vi "加标回收调试界面.vi"() -> ()   [LabVIEW 2016, in "质控单元V4.lvlib"]
uses:
  <vilib>/Utility/miscctls.llb/LVPointTypeDef.ctl
  <vilib>/Utility/miscctls.llb/LVPositionTypeDef.ctl
panel:
  in  "关闭":bool
  out "流程 2":T1 {"进样流程"."进样流程-进样"."步骤二："."功能" items=["加标", "进样", "排液", "搅拌", "定量", "延时"]; "进样流程"."进样流程-进样"."步骤一："."功能" items=["加标", "进样", "排液", "搅拌", "定量", "延时"]; "进样流程"."进样流程-进样"."步骤四："."功能" items=["加标", "进样", "排液", "搅拌", "定量", "延时"]; "进样流程"."进样流程-进样"."步骤三："."功能" items=["加标", "进样", "排液", "搅拌", "定量", "延时"]; "进样流程"."进样流程-进样"."步骤六："."功能" items=["加标", "进样", "排液", "搅拌", "定量", "延时"]; "进样流程"."进样流程-进样"."步骤五："."功能" items=["加标", "进样", "排液", "搅拌", "定量", "延时"]; "进样流程"."进样流程-进样"."步骤八："."功能" items=["加标", "进样", "排液", "搅拌", "定量", "延时"]; "进样流程"."进样流程-进样"."步骤七："."功能" items=["加标", "进样", "排液", "搅拌", "定量", "延时"]; "进样流程"."进样流程-进样"."步骤十："."功能" items=["加标", "进样", "排液", "搅拌", "定量", "延时"]; "进样流程"."进样流程-进样"."步骤九："."功能" items=["加标", "进样", "排液", "搅拌", "定量", "延时"]; "进样流程"."进样流程-润洗"."步骤二："."功能" items=["加标", "进样", "排液", "搅拌", "定量", "延时"]; "进样流程"."进样流程-润洗"."步骤一："."功能" items=["加标", "进样", "排液", "搅拌", "定量", "延时"]; "进样流程"."进样流程-润洗"."步骤四："."功能" items=["加标", "进样", "排液", "搅拌", "定量", "延时"]; "进样流程"."进样流程-润洗"."步骤三："."功能" items=["加标", "进样", "排液", "搅拌", "定量", "延时"]; "进样流程"."进样流程-润洗"."步骤六："."功能" items=["加标", "进样", "排液", "搅拌", "定量", "延时"]; "进样流程"."进样流程-润洗"."步骤五："."功能" items=["加标", "进样", "排液", "搅拌", "定量", "延时"]; "进样流程"."进样流程-润洗"."步骤八："."功能" items=["加标", "进样", "排液", "搅拌", "定量", "延时"]; "进样流程"."进样流程-润洗"."步骤七："."功能" items=["加标", "进样", "排液", "搅拌", "定量", "延时"]; "进样流程"."进样流程-润洗"."步骤十："."功能" items=["加标", "进样", "排液", "搅拌", "定量", "延时"]; "进样流程"."进样流程-润洗"."步骤九："."功能" items=["加标", "进样", "排液", "搅拌", "定量", "延时"]; "排液流程"."步骤二："."功能" items=["加标", "进样", "排液", "搅拌", "定量", "延时"]; "排液流程"."步骤一："."功能" items=["加标", "进样", "排液", "搅拌", "定量", "延时"]; "排液流程"."步骤四："."功能" items=["加标", "进样", "排液", "搅拌", "定量", "延时"]; "排液流程"."步骤三："."功能" items=["加标", "进样", "排液", "搅拌", "定量", "延时"]; "排液流程"."步骤六："."功能" items=["加标", "进样", "排液", "搅拌", "定量", "延时"]; "排液流程"."步骤五："."功能" items=["加标", "进样", "排液", "搅拌", "定量", "延时"]; "排液流程"."步骤八："."功能" items=["加标", "进样", "排液", "搅拌", "定量", "延时"]; "排液流程"."步骤七："."功能" items=["加标", "进样", "排液", "搅拌", "定量", "延时"]; "排液流程"."步骤十："."功能" items=["加标", "进样", "排液", "搅拌", "定量", "延时"]; "排液流程"."步骤九："."功能" items=["加标", "进样", "排液", "搅拌", "定量", "延时"]; "加标流程"."加标流程-加标"."步骤二："."功能" items=["加标", "进样", "排液", "搅拌", "定量", "延时"]; "加标流程"."加标流程-加标"."步骤一："."功能" items=["加标", "进样", "排液", "搅拌", "定量", "延时"]; "加标流程"."加标流程-加标"."步骤四："."功能" items=["加标", "进样", "排液", "搅拌", "定量", "延时"]; "加标流程"."加标流程-加标"."步骤三："."功能" items=["加标", "进样", "排液", "搅拌", "定量", "延时"]; "加标流程"."加标流程-加标"."步骤六："."功能" items=["加标", "进样", "排液", "搅拌", "定量", "延时"]; "加标流程"."加标流程-加标"."步骤五："."功能" items=["加标", "进样", "排液", "搅拌", "定量", "延时"]; "加标流程"."加标流程-加标"."步骤八："."功能" items=["加标", "进样", "排液", "搅拌", "定量", "延时"]; "加标流程"."加标流程-加标"."步骤七："."功能" items=["加标", "进样", "排液", "搅拌", "定量", "延时"]; "加标流程"."加标流程-加标"."步骤十："."功能" items=["加标", "进样", "排液", "搅拌", "定量", "延时"]; "加标流程"."加标流程-加标"."步骤九："."功能" items=["加标", "进样", "排液", "搅拌", "定量", "延时"]; "加标流程"."加标流程-定量"."步骤二："."功能" items=["加标", "进样", "排液", "搅拌", "定量", "延时"]; "加标流程"."加标流程-定量"."步骤一："."功能" items=["加标", "进样", "排液", "搅拌", "定量", "延时"]; "加标流程"."加标流程-定量"."步骤四："."功能" items=["加标", "进样", "排液", "搅拌", "定量", "延时"]; "加标流程"."加标流程-定量"."步骤三："."功能" items=["加标", "进样", "排液", "搅拌", "定量", "延时"]; "加标流程"."加标流程-定量"."步骤六："."功能" items=["加标", "进样", "排液", "搅拌", "定量", "延时"]; "加标流程"."加标流程-定量"."步骤五："."功能" items=["加标", "进样", "排液", "搅拌", "定量", "延时"]; "加标流程"."加标流程-定量"."步骤八："."功能" items=["加标", "进样", "排液", "搅拌", "定量", "延时"]; "加标流程"."加标流程-定量"."步骤七："."功能" items=["加标", "进样", "排液", "搅拌", "定量", "延时"]; "加标流程"."加标流程-定量"."步骤十："."功能" items=["加标", "进样", "排液", "搅拌", "定量", "延时"]; "加标流程"."加标流程-定量"."步骤九："."功能" items=["加标", "进样", "排液", "搅拌", "定量", "延时"]; "加标流程"."加标流程-进样"."步骤二："."功能" items=["加标", "进样", "排液", "搅拌", "定量", "延时"]; "加标流程"."加标流程-进样"."步骤一："."功能" items=["加标", "进样", "排液", "搅拌", "定量", "延时"]; "加标流程"."加标流程-进样"."步骤四："."功能" items=["加标", "进样", "排液", "搅拌", "定量", "延时"]; "加标流程"."加标流程-进样"."步骤三："."功能" items=["加标", "进样", "排液", "搅拌", "定量", "延时"]; "加标流程"."加标流程-进样"."步骤六："."功能" items=["加标", "进样", "排液", "搅拌", "定量", "延时"]; "加标流程"."加标流程-进样"."步骤五："."功能" items=["加标", "进样", "排液", "搅拌", "定量", "延时"]; "加标流程"."加标流程-进样"."步骤八："."功能" items=["加标", "进样", "排液", "搅拌", "定量", "延时"]; "加标流程"."加标流程-进样"."步骤七："."功能" items=["加标", "进样", "排液", "搅拌", "定量", "延时"]; "加标流程"."加标流程-进样"."步骤十："."功能" items=["加标", "进样", "排液", "搅拌", "定量", "延时"]; "加标流程"."加标流程-进样"."步骤九："."功能" items=["加标", "进样", "排液", "搅拌", "定量", "延时"]; "加标流程"."加标流程-润洗"."步骤二："."功能" items=["加标", "进样", "排液", "搅拌", "定量", "延时"]; "加标流程"."加标流程-润洗"."步骤一："."功能" items=["加标", "进样", "排液", "搅拌", "定量", "延时"]; "加标流程"."加标流程-润洗"."步骤四："."功能" items=["加标", "进样", "排液", "搅拌", "定量", "延时"]; "加标流程"."加标流程-润洗"."步骤三："."功能" items=["加标", "进样", "排液", "搅拌", "定量", "延时"]; "加标流程"."加标流程-润洗"."步骤六："."功能" items=["加标", "进样", "排液", "搅拌", "定量", "延时"]; "加标流程"."加标流程-润洗"."步骤五："."功能" items=["加标", "进样", "排液", "搅拌", "定量", "延时"]; "加标流程"."加标流程-润洗"."步骤八："."功能" items=["加标", "进样", "排液", "搅拌", "定量", "延时"]; "加标流程"."加标流程-润洗"."步骤七："."功能" items=["加标", "进样", "排液", "搅拌", "定量", "延时"]; "加标流程"."加标流程-润洗"."步骤十："."功能" items=["加标", "进样", "排液", "搅拌", "定量", "延时"]; "加标流程"."加标流程-润洗"."步骤九："."功能" items=["加标", "进样", "排液", "搅拌", "定量", "延时"]; "加标润洗流程"."步骤二："."功能" items=["加标", "进样", "排液", "搅拌", "定量", "延时"]; "加标润洗流程"."步骤一："."功能" items=["加标", "进样", "排液", "搅拌", "定量", "延时"]; "加标润洗流程"."步骤四："."功能" items=["加标", "进样", "排液", "搅拌", "定量", "延时"]; "加标润洗流程"."步骤三："."功能" items=["加标", "进样", "排液", "搅拌", "定量", "延时"]; "加标润洗流程"."步骤六："."功能" items=["加标", "进样", "排液", "搅拌", "定量", "延时"]; "加标润洗流程"."步骤五："."功能" items=["加标", "进样", "排液", "搅拌", "定量", "延时"]; "加标润洗流程"."步骤八："."功能" items=["加标", "进样", "排液", "搅拌", "定量", "延时"]; "加标润洗流程"."步骤七："."功能" items=["加标", "进样", "排液", "搅拌", "定量", "延时"]; "加标润洗流程"."步骤十："."功能" items=["加标", "进样", "排液", "搅拌", "定量", "延时"]; "加标润洗流程"."步骤九："."功能" items=["加标", "进样", "排液", "搅拌", "定量", "延时"]; "水样润洗流程"."步骤二："."功能" items=["加标", "进样", "排液", "搅拌", "定量", "延时"]; "水样润洗流程"."步骤一："."功能" items=["加标", "进样", "排液", "搅拌", "定量", "延时"]; "水样润洗流程"."步骤四："."功能" items=["加标", "进样", "排液", "搅拌", "定量", "延时"]; "水样润洗流程"."步骤三："."功能" items=["加标", "进样", "排液", "搅拌", "定量", "延时"]; "水样润洗流程"."步骤六："."功能" items=["加标", "进样", "排液", "搅拌", "定量", "延时"]; "水样润洗流程"."步骤五："."功能" items=["加标", "进样", "排液", "搅拌", "定量", "延时"]; "水样润洗流程"."步骤八："."功能" items=["加标", "进样", "排液", "搅拌", "定量", "延时"]; "水样润洗流程"."步骤七："."功能" items=["加标", "进样", "排液", "搅拌", "定量", "延时"]; "水样润洗流程"."步骤十："."功能" items=["加标", "进样", "排液", "搅拌", "定量", "延时"]; "水样润洗流程"."步骤九："."功能" items=["加标", "进样", "排液", "搅拌", "定量", "延时"]}
  in  "请选择模块":T2(radio)=enum."氨氮"
  in  "关于":bool
  in  "Tab Control 4":enum32{"参数"}(tab)
  out "剩余时间":string
  out "当前步骤":string
  out "当前流程":string
  out "告警状态":string
  out "液位状态":string
  out "运行状态":string
  out "通讯状态":bool caption="状态"
  in  "Tab Control 3":enum32{"参数设置", "单步调试", "流程写入"}(tab)
  in  "加标体积读取":bool
  in  "加标体积写入":bool
  in  "蠕动泵参数读取":bool
  in  "蠕动泵参数写入":bool
  in  "B":sgl
  in  "K":sgl
  in  "蠕动泵最小频率(Hz)":sgl
  in  "蠕动泵最大频率(Hz)":sgl
  in  "加标体积(mL)":sgl
  in  "注射泵系数读取":bool
  in  "注射泵系数写入":bool
  in  "质控类型":u16(ring) items=["固定站", "一体站"]
  in  "质控类型读取":bool
  in  "质控类型写入":bool
  in  "蠕动泵2停止":bool
  in  "蠕动泵2正转":bool
  in  "蠕动泵2反转":bool
  in  "蠕动泵1停止":bool
  in  "蠕动泵1正转":bool
  in  "蠕动泵1反转":bool
  in  "三通阀2打开":bool
  in  "三通阀2关闭":bool
  in  "三通阀1打开":bool
  in  "三通阀1关闭":bool
  in  "注射泵复位":bool
  in  "注射泵暂停":bool
  in  "注射泵注入量":sgl=1000.0 min=0 max=1000 format="%u μL"
  in  "注射泵注出量":sgl=1000.0 min=0 max=1000 format="%u μL"
  in  "注射泵注出":bool
  in  "注射泵注入":bool
  in  "三通阀打开":bool
  in  "三通阀关闭":bool
  in  "流程保存":bool
  in  "流程加载":bool
  in  "流程写入":bool
  in  "流程读取":bool
  in  "子流程":u16(ring) items=["润洗"]
  in  "主流程":T3(ring)
  in  "流程":T4 {"步骤二："."功能" items=["加标", "进样", "排液", "搅拌", "定量", "延时"]; "步骤四："."功能" items=["加标", "进样", "排液", "搅拌", "定量", "延时"]; "步骤六："."功能" items=["加标", "进样", "排液", "搅拌", "定量", "延时"]; "步骤八："."功能" items=["加标", "进样", "排液", "搅拌", "定量", "延时"]; "步骤十："."功能" items=["加标", "进样", "排液", "搅拌", "定量", "延时"]; "步骤一："."功能" items=["加标", "进样", "排液", "搅拌", "定量", "延时"]; "步骤三："."功能" items=["加标", "进样", "排液", "搅拌", "定量", "延时"]; "步骤五："."功能" items=["加标", "进样", "排液", "搅拌", "定量", "延时"]; "步骤七："."功能" items=["加标", "进样", "排液", "搅拌", "定量", "延时"]; "步骤九："."功能" items=["加标", "进样", "排液", "搅拌", "定量", "延时"]}
  in  "Tab Control 2":enum32{"参数"}(tab)
  in  "启动水样润洗流程":bool
  in  "启动进样流程":bool
  in  "启动加标流程":bool
  in  "启动排液流程":bool
  in  "停止所有流程":bool
  in  "启动加标润洗流程":bool
  in  "组合操作停止":bool
  in  "组合操作定量":bool
  in  "组合操作进空气":bool
  in  "组合操作排废液":bool
  in  "组合操作进水样":bool
  in  "清除告警":bool
  # "仪器状态"
  # "柱塞泵泵系数"
  # "柱塞泵"
  # "三通阀"
  # "泵阀"
  # "三通阀1"
  # "三通阀2"
  # "蠕动泵1"
  # "蠕动泵2"
  # "仪器端："
  # "PC端："
  # "组合步骤"
  # "测试流程"
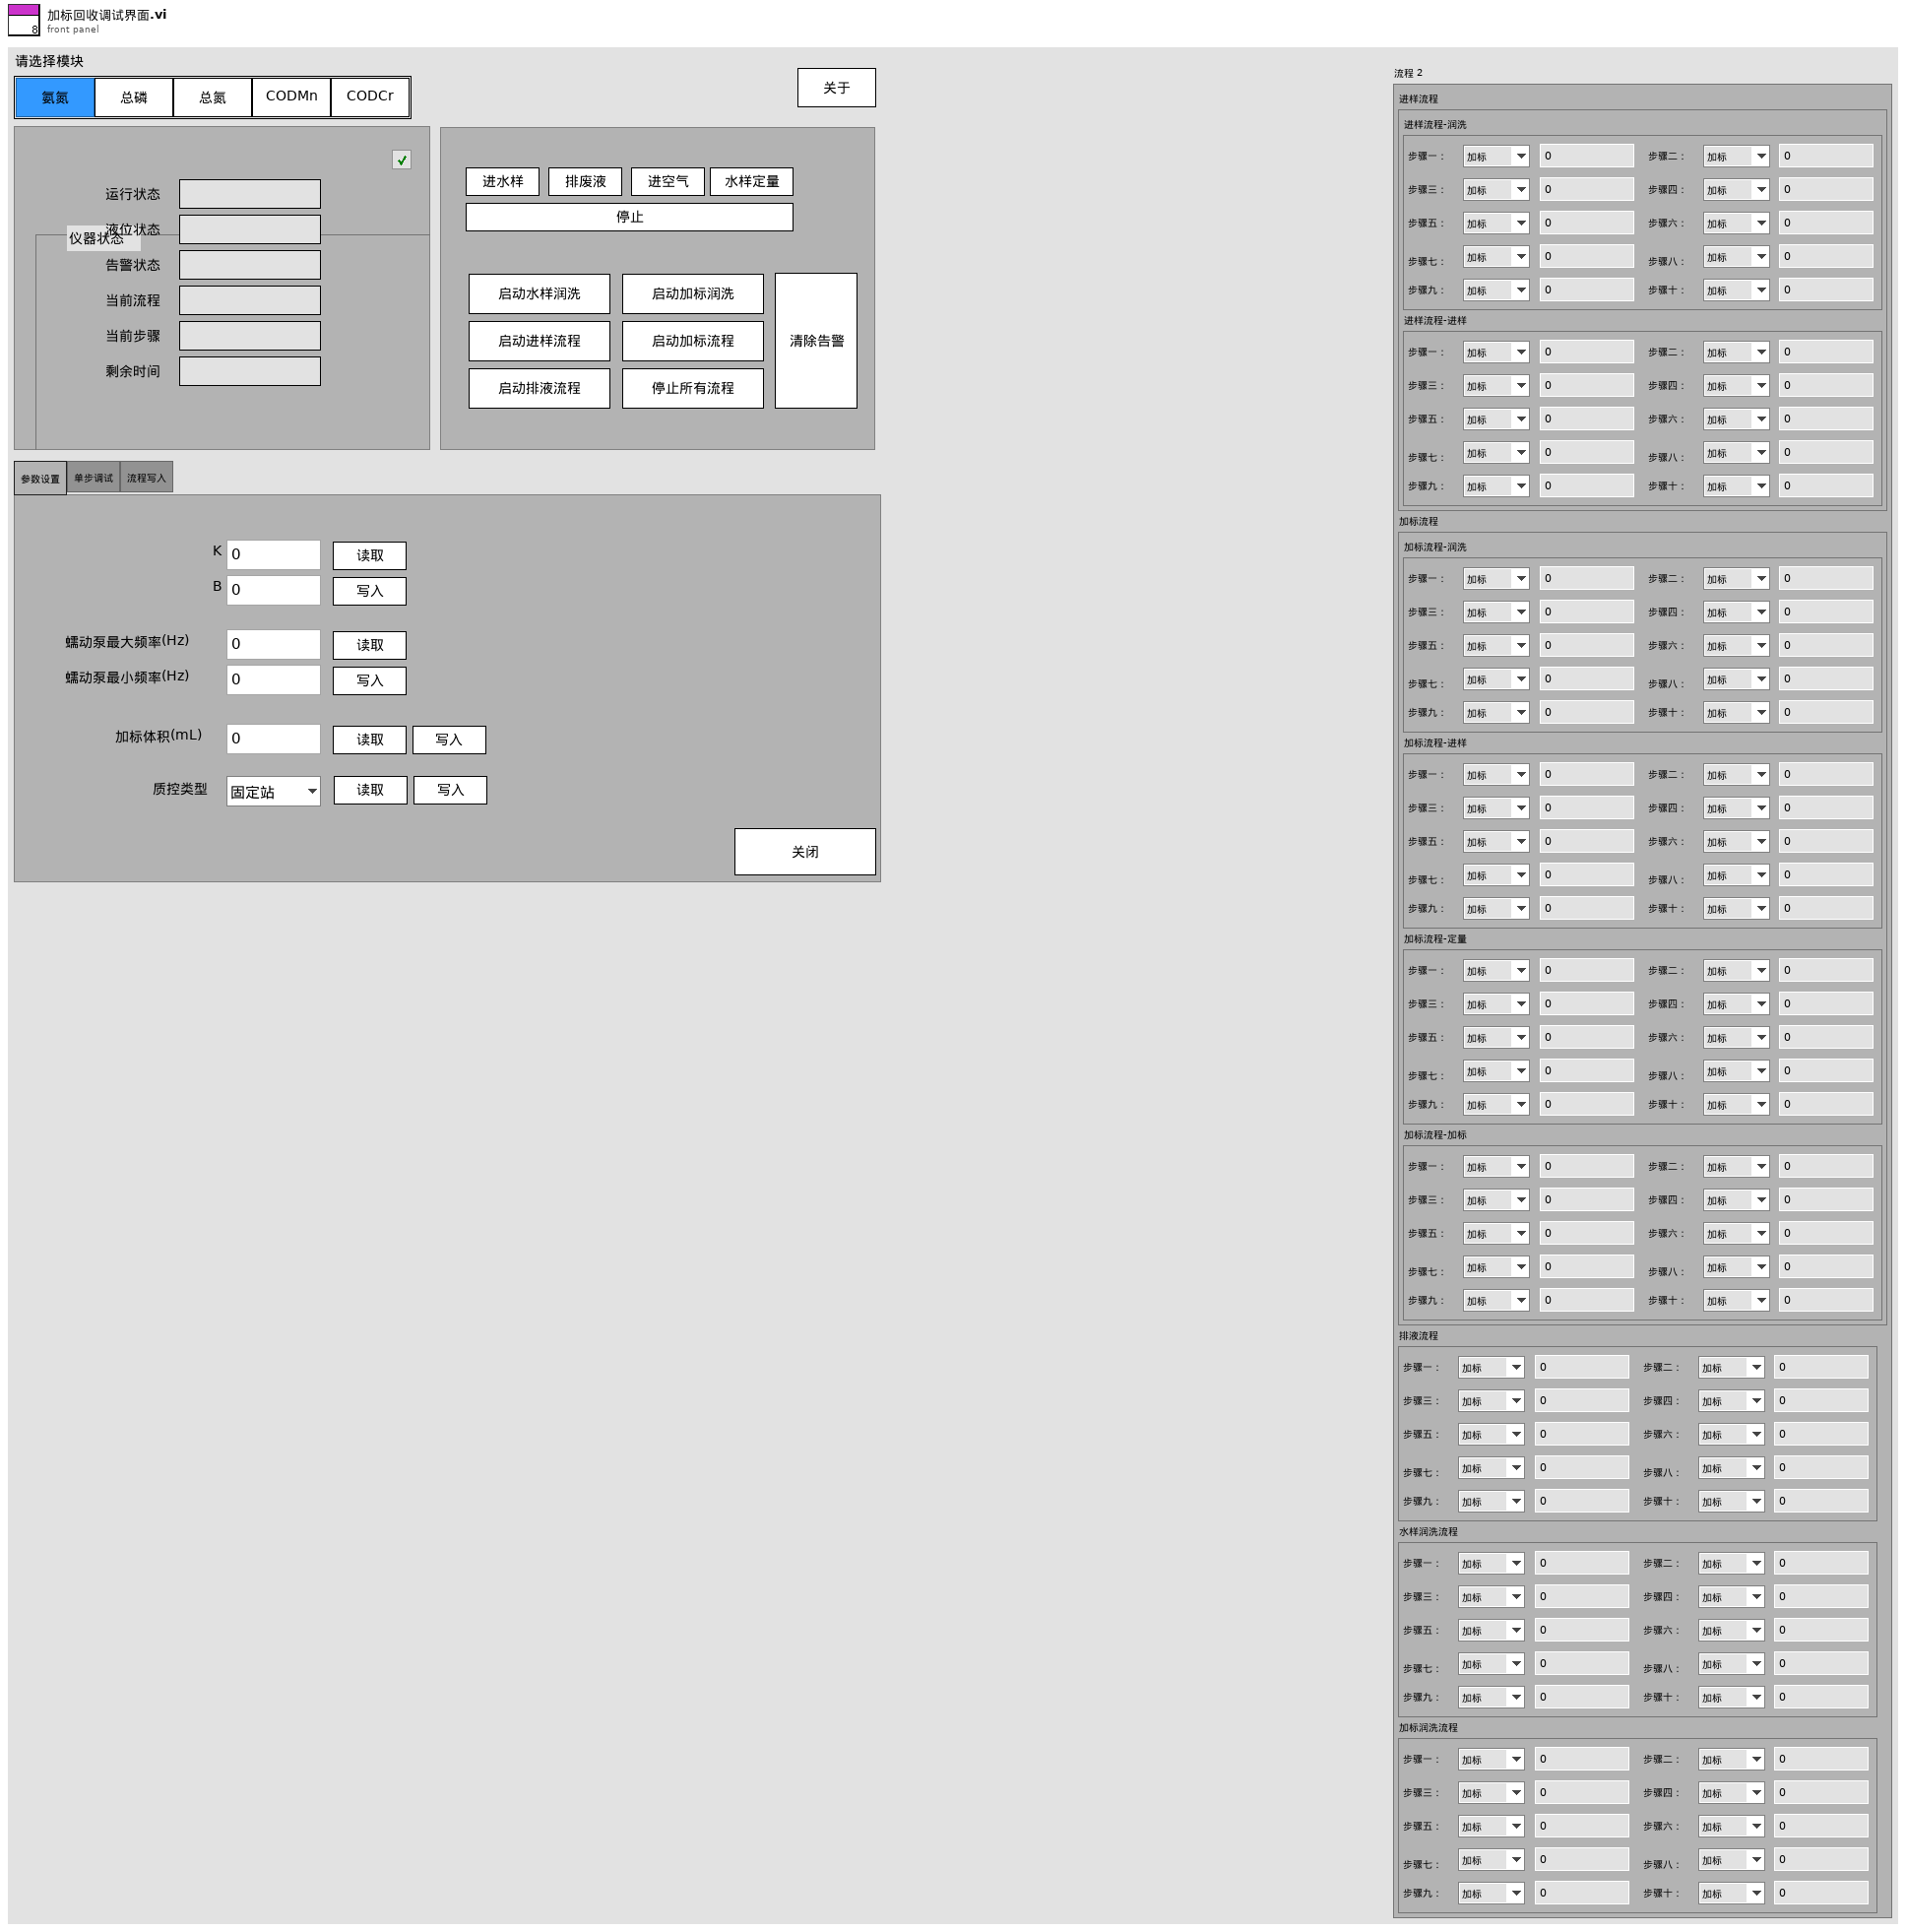
[diagram p1: front panel]
types:
  T1 = cluster{"进样流程":cluster{"进样流程-润洗":cluster{"步骤一：":cluster{"功能":u16, "值":sgl}, "步骤二：":cluster{"功能":u16, "值":sgl}, "步骤三：":cluster{"功能":u16, "值":sgl}, "步骤四：":cluster{"功能":u16, "值":sgl}, "步骤五：":cluster{"功能":u16, "值":sgl}, "步骤六：":cluster{"功能":u16, "值":sgl}, "步骤七：":cluster{"功能":u16, "值":sgl}, "步骤八：":cluster{"功能":u16, "值":sgl}, "步骤九：":cluster{"功能":u16, "值":sgl}, "步骤十：":cluster{"功能":u16, "值":sgl}}, "进样流程-进样":cluster{"步骤一：":cluster{"功能":u16, "值":sgl}, "步骤二：":cluster{"功能":u16, "值":sgl}, "步骤三：":cluster{"功能":u16, "值":sgl}, "步骤四：":cluster{"功能":u16, "值":sgl}, "步骤五：":cluster{"功能":u16, "值":sgl}, "步骤六：":cluster{"功能":u16, "值":sgl}, "步骤七：":cluster{"功能":u16, "值":sgl}, "步骤八：":cluster{"功能":u16, "值":sgl}, "步骤九：":cluster{"功能":u16, "值":sgl}, "步骤十：":cluster{"功能":u16, "值":sgl}}}, "加标流程":cluster{"加标流程-润洗":cluster{"步骤一：":cluster{"功能":u16, "值":sgl}, "步骤二：":cluster{"功能":u16, "值":sgl}, "步骤三：":cluster{"功能":u16, "值":sgl}, "步骤四：":cluster{"功能":u16, "值":sgl}, "步骤五：":cluster{"功能":u16, "值":sgl}, "步骤六：":cluster{"功能":u16, "值":sgl}, "步骤七：":cluster{"功能":u16, "值":sgl}, "步骤八：":cluster{"功能":u16, "值":sgl}, "步骤九：":cluster{"功能":u16, "值":sgl}, "步骤十：":cluster{"功能":u16, "值":sgl}}, "加标流程-进样":cluster{"步骤一：":cluster{"功能":u16, "值":sgl}, "步骤二：":cluster{"功能":u16, "值":sgl}, "步骤三：":cluster{"功能":u16, "值":sgl}, "步骤四：":cluster{"功能":u16, "值":sgl}, "步骤五：":cluster{"功能":u16, "值":sgl}, "步骤六：":cluster{"功能":u16, "值":sgl}, "步骤七：":cluster{"功能":u16, "值":sgl}, "步骤八：":cluster{"功能":u16, "值":sgl}, "步骤九：":cluster{"功能":u16, "值":sgl}, "步骤十：":cluster{"功能":u16, "值":sgl}}, "加标流程-定量":cluster{"步骤一：":cluster{"功能":u16, "值":sgl}, "步骤二：":cluster{"功能":u16, "值":sgl}, "步骤三：":cluster{"功能":u16, "值":sgl}, "步骤四：":cluster{"功能":u16, "值":sgl}, "步骤五：":cluster{"功能":u16, "值":sgl}, "步骤六：":cluster{"功能":u16, "值":sgl}, "步骤七：":cluster{"功能":u16, "值":sgl}, "步骤八：":cluster{"功能":u16, "值":sgl}, "步骤九：":cluster{"功能":u16, "值":sgl}, "步骤十：":cluster{"功能":u16, "值":sgl}}, "加标流程-加标":cluster{"步骤一：":cluster{"功能":u16, "值":sgl}, "步骤二：":cluster{"功能":u16, "值":sgl}, "步骤三：":cluster{"功能":u16, "值":sgl}, "步骤四：":cluster{"功能":u16, "值":sgl}, "步骤五：":cluster{"功能":u16, "值":sgl}, "步骤六：":cluster{"功能":u16, "值":sgl}, "步骤七：":cluster{"功能":u16, "值":sgl}, "步骤八：":cluster{"功能":u16, "值":sgl}, "步骤九：":cluster{"功能":u16, "值":sgl}, "步骤十：":cluster{"功能":u16, "值":sgl}}}, "排液流程":cluster{"步骤一：":cluster{"功能":u16, "值":sgl}, "步骤二：":cluster{"功能":u16, "值":sgl}, "步骤三：":cluster{"功能":u16, "值":sgl}, "步骤四：":cluster{"功能":u16, "值":sgl}, "步骤五：":cluster{"功能":u16, "值":sgl}, "步骤六：":cluster{"功能":u16, "值":sgl}, "步骤七：":cluster{"功能":u16, "值":sgl}, "步骤八：":cluster{"功能":u16, "值":sgl}, "步骤九：":cluster{"功能":u16, "值":sgl}, "步骤十：":cluster{"功能":u16, "值":sgl}}, "水样润洗流程":cluster{"步骤一：":cluster{"功能":u16, "值":sgl}, "步骤二：":cluster{"功能":u16, "值":sgl}, "步骤三：":cluster{"功能":u16, "值":sgl}, "步骤四：":cluster{"功能":u16, "值":sgl}, "步骤五：":cluster{"功能":u16, "值":sgl}, "步骤六：":cluster{"功能":u16, "值":sgl}, "步骤七：":cluster{"功能":u16, "值":sgl}, "步骤八：":cluster{"功能":u16, "值":sgl}, "步骤九：":cluster{"功能":u16, "值":sgl}, "步骤十：":cluster{"功能":u16, "值":sgl}}, "加标润洗流程":cluster{"步骤一：":cluster{"功能":u16, "值":sgl}, "步骤二：":cluster{"功能":u16, "值":sgl}, "步骤三：":cluster{"功能":u16, "值":sgl}, "步骤四：":cluster{"功能":u16, "值":sgl}, "步骤五：":cluster{"功能":u16, "值":sgl}, "步骤六：":cluster{"功能":u16, "值":sgl}, "步骤七：":cluster{"功能":u16, "值":sgl}, "步骤八：":cluster{"功能":u16, "值":sgl}, "步骤九：":cluster{"功能":u16, "值":sgl}, "步骤十：":cluster{"功能":u16, "值":sgl}}}
  T2 = enum32{"未选择", "氨氮", "总磷", "总氮", "CODMn", "CODCr", "氨氮总磷", "总磷总氮"}
  T3 = enum16{"水样润洗流程", "加标润洗流程", "进样流程", "加标流程", "排液流程"}
  T4 = cluster{"步骤一：":cluster{"功能":u16, "值":sgl}, "步骤二：":cluster{"功能":u16, "值":sgl}, "步骤三：":cluster{"功能":u16, "值":sgl}, "步骤四：":cluster{"功能":u16, "值":sgl}, "步骤五：":cluster{"功能":u16, "值":sgl}, "步骤六：":cluster{"功能":u16, "值":sgl}, "步骤七：":cluster{"功能":u16, "值":sgl}, "步骤八：":cluster{"功能":u16, "值":sgl}, "步骤九：":cluster{"功能":u16, "值":sgl}, "步骤十：":cluster{"功能":u16, "值":sgl}}
  T5 = typedef "LVPositionTypeDef.ctl" = cluster{"Left":i32, "Top":i32}
  T6 = typedef "LVPointTypeDef.ctl" = cluster{"Horizontal":i16, "Vertical":i16}
  T7 = typedef "质控单元V4.lvlib/质控slave id.ctl" = enum16{"null", "氨氮", "总磷", "总氮", "CODMn", "CODCr"}
  T8 = typedef "质控单元V4.lvlib/质控注射泵操作.ctl" = enum16{"打开三通阀", "关闭三通阀", "注射泵吸入", "注射泵排出", "注射泵暂停", "注射泵复位"}
  T9 = typedef "质控单元V4.lvlib/质控组合命令区.ctl" = enum16{"停止", "进水样", "排废液", "进空气（搅拌）", "定量（反转定量）"}
  T10 = typedef "质控单元V4.lvlib/质控流程控制.ctl" = enum16{"待机", "启动进样流程", "启动加标流程", "启动排液流程", "启动水样润洗流程", "启动加标润洗流程", "停止流程"}
  T11 = typedef "质控单元V4.lvlib/质控仪器状态显示.ctl" = cluster{"运行模式":string, "运行状态":string, "液位状态":string, "告警状态":string, "当前流程":string, "当前步骤":string, "剩余时间":string}
  T12 = typedef "质控单元V4.lvlib/质控型号.ctl" = u16
  T13 = typedef "质控单元V4.lvlib/质控蠕动泵操作.ctl" = u16
  T14 = typedef "LVRectTypeDef.ctl" = cluster{"Left":i16, "Top":i16, "Right":i16, "Bottom":i16}
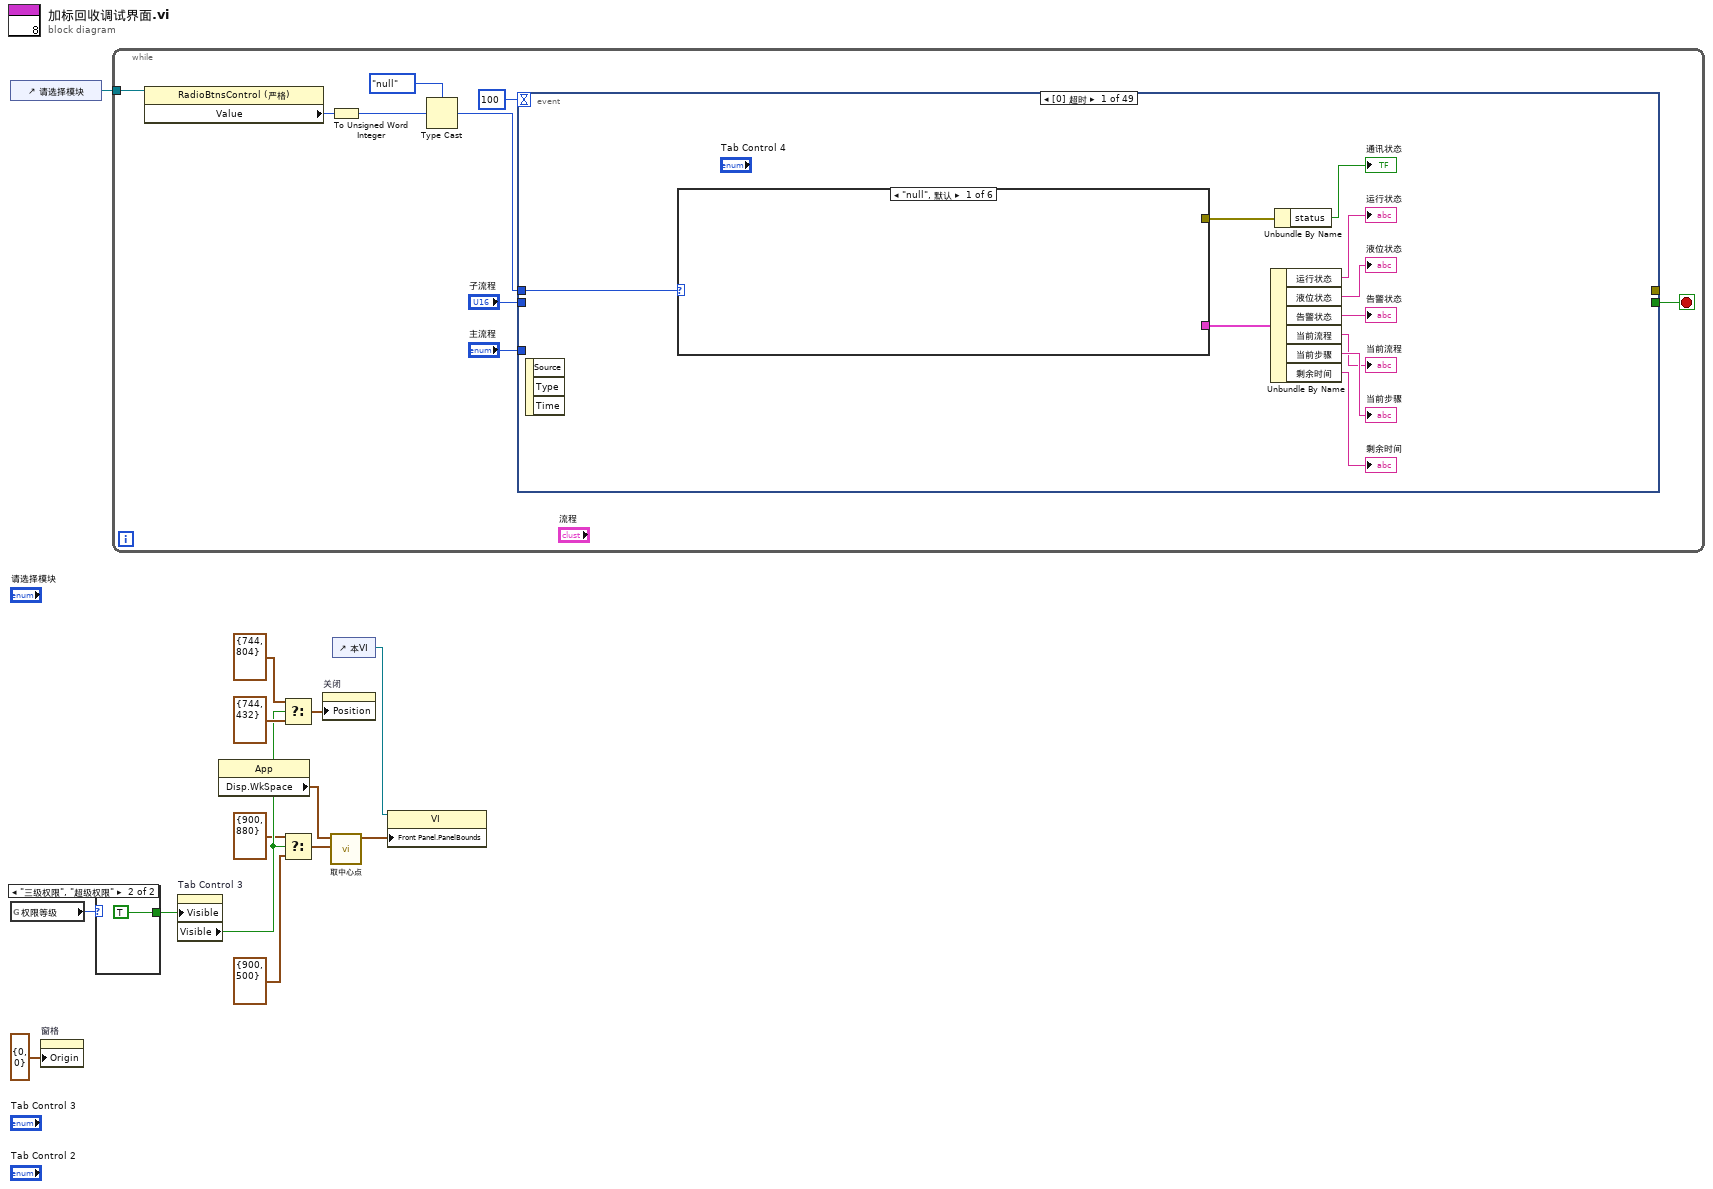
[diagram p0: block diagram]
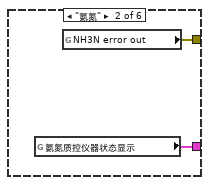
[diagram p3: hidden frame]
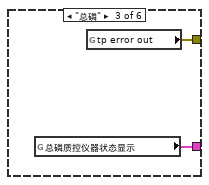
[diagram p4: hidden frame]
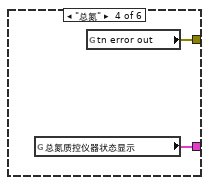
[diagram p5: hidden frame]
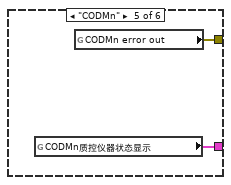
[diagram p6: hidden frame]
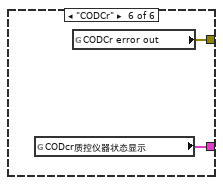
[diagram p7: hidden frame]
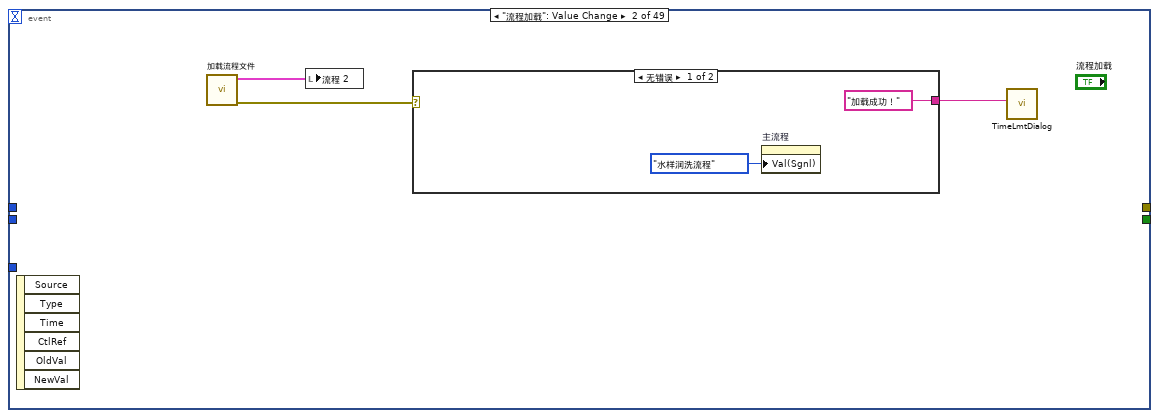
[diagram p8: hidden frame]
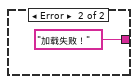
[diagram p9: hidden frame]
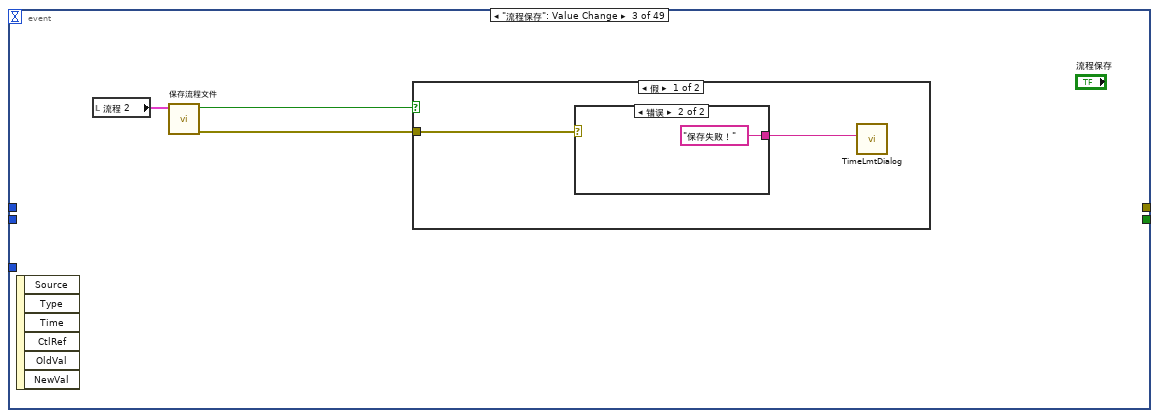
[diagram p10: hidden frame]
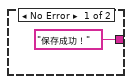
[diagram p11: hidden frame]
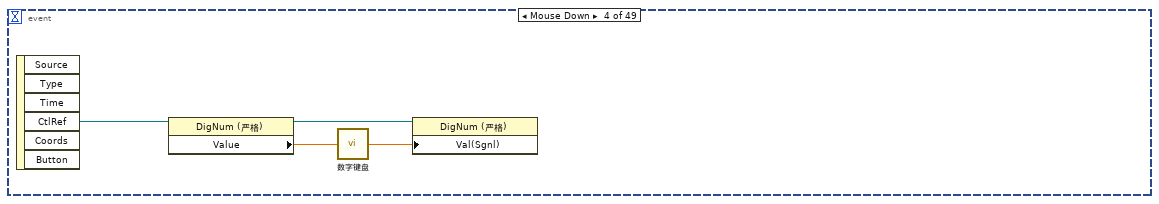
[diagram p13: hidden frame]
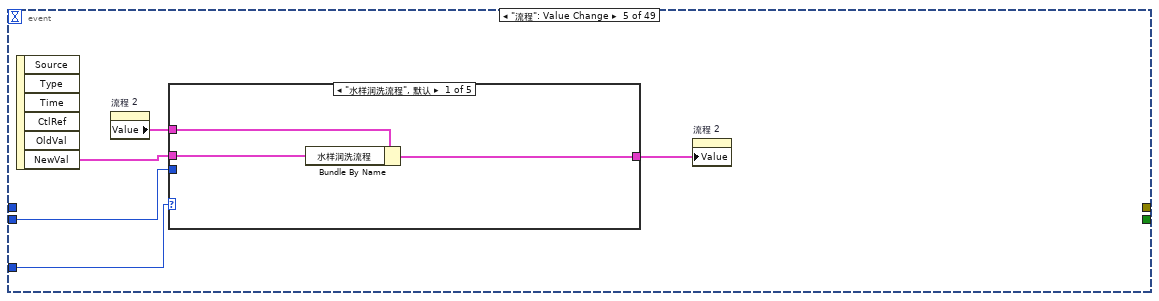
[diagram p14: hidden frame]
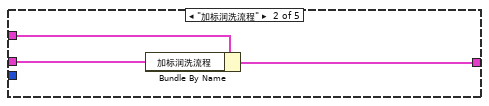
[diagram p15: hidden frame]
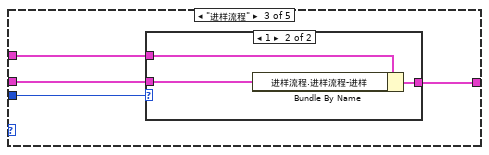
[diagram p16: hidden frame]
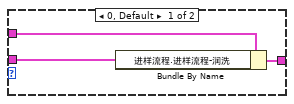
[diagram p17: hidden frame]
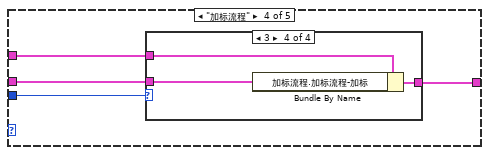
[diagram p18: hidden frame]
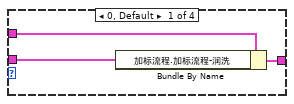
[diagram p19: hidden frame]
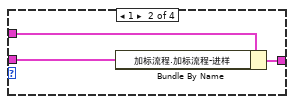
[diagram p20: hidden frame]
diagram:
  n1 = control-ref of="请选择模块"() -> (w13:refnum<vi>)
  n2 = global read "ZK非断电保存全局变量.vi" "权限等级"() -> (w2:enum16{"一级权限", "二级权限", "三级权限", "超级权限"})
  n3 = property on="窗格" class="Pane"("Origin"=T6 {"Horizontal"=0, "Vertical"=0} ("原点")) -> ()  [unwired: 2 in, 2 out]
  n4 = case shown="\"三级权限\", \"超级权限\"" w2 {
    tunnel: [_ TRUE] -> w1
    frame "一级权限", Default {
    }
    frame "三级权限", "超级权限" {
    }
  }
  n5 = while {
    tunnel: w13 -> [w22]
    stop <- w24 stop-if-true
    n6 = property class="RadioBtnsControl (严格)"(reference=w22) -> ("Value"=w19:T2)  [unwired: 1 in, 2 out]
    n7 = To Unsigned Word Integer(number=w19) -> (unsigned 16bit integer=w18:u16)
    n8 = Type Cast(type=质控slave_id."null" ("请选择模块"), x=w18) -> (*(type *) &x=w20:T7)
    n9 = event shown="[0] 超时" {
      selector: _ -> [_ _ _ _ _ _ _ _ _ _ _ _ _ _ _ _ _ _ _ _ _ _ _ _ _ _ _ _ _ _ _ _ _ _ _ _ _ _ _ _ _ _ _ _ _ _ _ _ _]
      dyn-events: _ -> [_ _ _ _ _ _ _ _ _ _ _ _ _ _ _ _ _ _ _ _ _ _ _ _ _ _ _ _ _ _ _ _ _ _ _ _ _ _ _ _ _ _ _ _ _ _ _ _ _]
      timeout: 100 -> [_ _ _ _ _ _ _ _ _ _ _ _ _ _ _ _ _ _ _ _ _ _ _ _ _ _ _ _ _ _ _ _ _ _ _ _ _ _ _ _ _ _ _ _ _ _ _ _ _]
      tunnel: [_ _ _ _ _ _ _ _ _ _ _ _ _ TRUE _ _ _ _ _ _ _ _ _ _ _ _ _ _ _ _ _ _ _ _ _ _ _ _ _ _ _ _ _ _ _ _ _ _ _] -> w24
      tunnel: [_ _ _ _ _ _ _ _ _ _ w175 w179 w184 _ _ _ w198 w203 w210 w213 w219 w223 w226 w231 w241 w251 w255 w259 w262 w266 w270 w274 w279 w283 w287 w291 w295 w299 w303 w307 w311 w315 w319 w323 w327 w331 w335 w339 w343] -> _
      tunnel: w20 -> [w27 _ _ _ _ w105 w108 _ _ w173 w174 w178 w182 _ _ _ w196 w201 w206 w211 w216 w220 w224 w228 w234 w245 w252 w256 w260 w264 w268 w272 w276 w280 w284 w288 w292 w296 w300 w304 w308 w312 w316 w320 w324 w328 w332 w336 w340]
      tunnel: "子流程" -> [_ _ _ _ w64 _ _ w114 _ _ _ _ _ _ _ _ _ _ _ _ _ _ _ _ _ _ _ _ _ _ _ _ _ _ _ _ _ _ _ _ _ _ _ _ _ _ _ _ _]
      tunnel: "主流程" -> [_ _ _ _ w65 _ _ _ w146 _ _ _ _ _ _ _ _ _ _ _ _ _ _ _ _ _ _ _ _ _ _ _ _ _ _ _ _ _ _ _ _ _ _ _ _ _ _ _ _]
      event Timeout {
        n10 = event-data() -> ()  [unwired: 1 in, 3 out]
        n11 = case shown="\"null\", 默认" w27 {
          tunnel: [_ w36 w38 w40 w42 w44] -> w34
          tunnel: [_ w35 w37 w39 w41 w43] -> w26
          frame "null", Default {
          }
          frame "氨氮" {
            n12 = global read "ZK非断电保存全局变量.vi" "氨氮质控仪器状态显示"() -> (w36:T11)
            n13 = global read "ZK非断电保存全局变量.vi" "NH3N error out"() -> (w35:errorcluster)
          }
          frame "总磷" {
            n14 = global read "ZK非断电保存全局变量.vi" "总磷质控仪器状态显示"() -> (w38:T11)
            n15 = global read "ZK非断电保存全局变量.vi" "tp error out"() -> (w37:errorcluster)
          }
          frame "总氮" {
            n16 = global read "ZK非断电保存全局变量.vi" "总氮质控仪器状态显示"() -> (w40:T11)
            n17 = global read "ZK非断电保存全局变量.vi" "tn error out"() -> (w39:errorcluster)
          }
          frame "CODMn" {
            n18 = global read "ZK非断电保存全局变量.vi" "CODMn质控仪器状态显示"() -> (w42:T11)
            n19 = global read "ZK非断电保存全局变量.vi" "CODMn error out"() -> (w41:errorcluster)
          }
          frame "CODCr" {
            n20 = global read "ZK非断电保存全局变量.vi" "CODcr质控仪器状态显示"() -> (w44:T11)
            n21 = global read "ZK非断电保存全局变量.vi" "CODCr error out"() -> (w43:errorcluster)
          }
        }
        n22 = Unbundle By Name(w34) -> ("运行状态"=→"运行状态":string, "液位状态"=→"液位状态":string, "告警状态"=→"告警状态":string, "当前流程"=→"当前流程":string, "当前步骤"=→"当前步骤":string, "剩余时间"=→"剩余时间":string)
        n23 = Unbundle By Name(w26) -> ("status"=→"通讯状态":bool)
      }
      event "流程加载": Value Change {
        n24 = event-data() -> ()  [unwired: 1 in, 6 out]
        n25 = call "加载流程文件.vi"() -> ("错误输出"=w46:errorcluster, "流程"=w47:T1)  [unwired: 10 in]
        n26 = local write "流程 2"(w47) -> ()
        n27 = case shown="无错误" w46 {
          tunnel: ["加载成功！" "加载失败！"] -> w45
          frame No Error {
            n28 = property on="主流程" class="Enum (严格)"("Val(Sgnl)"=T3."水样润洗流程" ("值(信号)")) -> ()  [unwired: 2 in, 2 out]
          }
          frame Error {
          }
        }
        n29 = call "TimeLmtDialog.vi"("Infoin"=w45) -> ()  [unwired: 11 in]
      }
      event "流程保存": Value Change {
        n30 = event-data() -> ()  [unwired: 1 in, 6 out]
        n31 = local read "流程 2"() -> (w53:T1)
        n32 = call "保存流程文件.vi"("流程"=w53) -> ("错误输出"=w52:errorcluster, "cancelled"=w51:bool)  [unwired: 9 in]
        n33 = case shown="假" w51 {
          tunnel: w52 -> [w54 _]
          frame False {
            n34 = case shown="错误" w54 {
              tunnel: ["保存成功！" "保存失败！"] -> w55
              frame No Error {
              }
              frame Error {
              }
            }
            n35 = call "TimeLmtDialog.vi"("Infoin"=w55) -> ()  [unwired: 11 in]
          }
          frame True {
          }
        }
      }
      event "流程.步骤一：.值", "流程.步骤二：.值", "流程.步骤三：.值", "流程.步骤四：.值", "流程.步骤五：.值", "流程.步骤六：.值", "流程.步骤七：.值", "流程.步骤八：.值", "流程.步骤九：.值", "流程.步骤十：.值": Mouse Down {
        n36 = event-data() -> ("CtlRef"=w58:refnum<vi>)  [unwired: 1 in, 5 out]
        n37 = property class="DigNum (严格)"(reference=w58) -> (reference out=w61:refnum<vi>, "Value"=w59:sgl)  [unwired: 1 in, 1 out]
        n38 = call "数字键盘.vi"("OldNumber"=w59) -> ("NewNumber"=w60:sgl)
        n39 = property class="DigNum (严格)"(reference=w61, "Val(Sgnl)"=w60) -> ()  [unwired: 1 in, 2 out]
      }
      event "流程": Value Change {
        n40 = event-data() -> ("NewVal"=w63:T4)  [unwired: 1 in, 5 out]
        n41 = property on="流程 2" class="Clust (严格)"() -> ("Value"=w66:T1)  [unwired: 2 in, 2 out]
        n42 = case shown="\"水样润洗流程\", 默认" w65 {
          tunnel: w66 -> [w69 w72 w75 w85 w101]
          tunnel: w64 -> [_ _ w76 w86 _]
          tunnel: w63 -> [w68 w71 w74 w83 w100]
          tunnel: [w67 w70 w73 w84 w99] -> w62
          frame "水样润洗流程", Default {
            n43 = Bundle By Name(cluster=w69, "水样润洗流程"=w68) -> (w67:T1)
          }
          frame "加标润洗流程" {
            n44 = Bundle By Name(cluster=w72, "加标润洗流程"=w71) -> (w70:T1)
          }
          frame "进样流程" {
            n45 = case shown="1" w76 {
              tunnel: w75 -> [w79 w82]
              tunnel: w74 -> [w78 w81]
              tunnel: [w77 w80] -> w73
              frame 0, Default {
                n46 = Bundle By Name(cluster=w79, "进样流程.进样流程-润洗"=w78) -> (w77:T1)
              }
              frame 1 {
                n47 = Bundle By Name(cluster=w82, "进样流程.进样流程-进样"=w81) -> (w80:T1)
              }
            }
          }
          frame "加标流程" {
            n48 = case shown="3" w86 {
              tunnel: w85 -> [w89 w92 w94 w98]
              tunnel: [w88 w90 w93 w96] -> w84
              tunnel: w83 -> [w87 w91 w95 w97]
              frame 0, Default {
                n49 = Bundle By Name(cluster=w89, "加标流程.加标流程-润洗"=w87) -> (w88:T1)
              }
              frame 1 {
                n50 = Bundle By Name(cluster=w92, "加标流程.加标流程-进样"=w91) -> (w90:T1)
              }
              frame 2 {
                n51 = Bundle By Name(cluster=w94, "加标流程.加标流程-定量"=w95) -> (w93:T1)
              }
              frame 3 {
                n52 = Bundle By Name(cluster=w98, "加标流程.加标流程-加标"=w97) -> (w96:T1)
              }
            }
          }
          frame "排液流程" {
            n53 = Bundle By Name(cluster=w101, "排液流程"=w100) -> (w99:T1)
          }
        }
        n54 = property on="流程 2" class="Clust (严格)"("Value"=w62) -> ()  [unwired: 2 in, 2 out]
      }
      event "流程读取": Value Change {
        n55 = event-data() -> ()  [unwired: 1 in, 6 out]
        n56 = call "ZK流程读取.vi"("是否启用通讯通知"=TRUE, "Slave ID"=w105) -> ("error out"=w102:errorcluster, "流程"=→"流程 2":T1)  [unwired: 8 in]
        n57 = case shown="无错误" w102 {
          frame No Error {
            n58 = property on="主流程" class="Enum (严格)"("Val(Sgnl)"=T3."水样润洗流程" ("值(信号)")) -> ()  [unwired: 2 in, 2 out]
          }
          frame Error {
          }
        }
      }
      event "流程写入": Value Change {
        n59 = event-data() -> ()  [unwired: 1 in, 6 out]
        n60 = property on="流程 2" class="Clust (严格)"() -> ("Value"=w109:T1)  [unwired: 2 in, 2 out]
        n61 = call "ZK流程写入.vi"("是否启用通讯通知"=TRUE, "流程"=w109, "Slave ID"=w108) -> ()  [unwired: 8 in, 1 out]
      }
      event "主流程": Value Change {
        n62 = event-data() -> ("NewVal"=w110:T3)  [unwired: 1 in, 5 out]
        n63 = local read "流程 2"() -> (w115:T1)
        n64 = case shown="\"排液流程\"" w110 {
          tunnel: w115 -> [w118 w121 w124 w132 w144]
          tunnel: w114 -> [_ _ w125 w133 _]
          tunnel: [w117 w120 w123 w131 w143] -> w113
          tunnel: [string[] ["润洗"] ("字符串[]") string[] ["润洗"] ("字符串[]") string[] ["润洗", "进样"] ("字符串[]") string[] ["润洗", "进样", "定量", "加标"] ("字符串[]") string[] ["排液"] ("字符串[]")] -> w112
          frame "水样润洗流程", Default {
            n65 = Unbundle By Name(w118) -> ("水样润洗流程"=w117:T4)
          }
          frame "加标润洗流程" {
            n66 = Unbundle By Name(w121) -> ("加标润洗流程"=w120:T4)
          }
          frame "进样流程" {
            n67 = case shown="0, 默认" w125 {
              tunnel: w124 -> [w127 w129]
              tunnel: [w126 w128] -> w123
              frame 0, Default {
                n68 = Unbundle By Name(w127) -> ("进样流程.进样流程-润洗"=w126:T4)
              }
              frame 1 {
                n69 = Unbundle By Name(w129) -> ("进样流程.进样流程-进样"=w128:T4)
              }
            }
          }
          frame "加标流程" {
            n70 = case shown="3" w133 {
              tunnel: w132 -> [w135 w137 w139 w141]
              tunnel: [w134 w136 w138 w140] -> w131
              frame 0, Default {
                n71 = Unbundle By Name(w135) -> ("加标流程.加标流程-润洗"=w134:T4)
              }
              frame 1 {
                n72 = Unbundle By Name(w137) -> ("加标流程.加标流程-进样"=w136:T4)
              }
              frame 2 {
                n73 = Unbundle By Name(w139) -> ("加标流程.加标流程-定量"=w138:T4)
              }
              frame 3 {
                n74 = Unbundle By Name(w141) -> ("加标流程.加标流程-加标"=w140:T4)
              }
            }
          }
          frame "排液流程" {
            n75 = Unbundle By Name(w144) -> ("排液流程"=w143:T4)
          }
        }
        n76 = local write "流程"(w113) -> ()
        n77 = property on="子流程" class="Ring (严格)"("Strings []"=w112, "Value"=0) -> ()  [unwired: 2 in, 2 out]
      }
      event "子流程": Value Change {
        n78 = event-data() -> ("NewVal"=w145:u16)  [unwired: 1 in, 5 out]
        n79 = local read "流程 2"() -> (w148:T1)
        n80 = case shown="\"排液流程\"" w146 {
          tunnel: w148 -> [w150 w152 w154 w161 w172]
          tunnel: w145 -> [_ _ w155 w162 _]
          tunnel: [w149 w151 w153 w160 w171] -> w147
          frame "水样润洗流程", Default {
            n81 = Unbundle By Name(w150) -> ("水样润洗流程"=w149:T4)
          }
          frame "加标润洗流程" {
            n82 = Unbundle By Name(w152) -> ("加标润洗流程"=w151:T4)
          }
          frame "进样流程" {
            n83 = case shown="0, 默认" w155 {
              tunnel: w154 -> [w157 w159]
              tunnel: [w156 w158] -> w153
              frame 0, Default {
                n84 = Unbundle By Name(w157) -> ("进样流程.进样流程-润洗"=w156:T4)
              }
              frame 1 {
                n85 = Unbundle By Name(w159) -> ("进样流程.进样流程-进样"=w158:T4)
              }
            }
          }
          frame "加标流程" {
            n86 = case shown="3" w162 {
              tunnel: w161 -> [w164 w166 w168 w170]
              tunnel: [w163 w165 w167 w169] -> w160
              frame 0, Default {
                n87 = Unbundle By Name(w164) -> ("加标流程.加标流程-润洗"=w163:T4)
              }
              frame 1 {
                n88 = Unbundle By Name(w166) -> ("加标流程.加标流程-进样"=w165:T4)
              }
              frame 2 {
                n89 = Unbundle By Name(w168) -> ("加标流程.加标流程-定量"=w167:T4)
              }
              frame 3 {
                n90 = Unbundle By Name(w170) -> ("加标流程.加标流程-加标"=w169:T4)
              }
            }
          }
          frame "排液流程" {
            n91 = Unbundle By Name(w172) -> ("排液流程"=w171:T4)
          }
        }
        n92 = local write "流程"(w147) -> ()
      }
      event "关于": Value Change {
        n93 = event-data() -> ()  [unwired: 1 in, 6 out]
        n94 = call "质控关于.vi"("Slave ID"=w173) -> ()  [unwired: 11 in]
      }
      event "质控类型读取": Value Change {
        n95 = event-data() -> ()  [unwired: 1 in, 6 out]
        n96 = call "ZK型号读取.vi"("是否启用通讯通知"=TRUE, "Slave ID"=w174) -> ("error out"=w175:errorcluster, "质控型号"=w176:T12)  [unwired: 8 in]
        n97 = local write "质控类型"(w176) -> ()
      }
      event "质控类型写入": Value Change {
        n98 = event-data() -> ()  [unwired: 1 in, 6 out]
        n99 = call "ZK型号写入.vi"("是否启用通讯通知"=TRUE, "质控型号"="质控类型", "Slave ID"=w178) -> ("error out"=w179:errorcluster)  [unwired: 8 in]
      }
      event "清除告警": Value Change {
        n100 = event-data() -> ()  [unwired: 1 in, 6 out]
        n101 = call "ZK报警清除.vi"("是否启用通讯通知"=TRUE, "Slave ID"=w182) -> ("error out"=w184:errorcluster)  [unwired: 9 in]
      }
      event Panel Close; "关闭": Value Change {
        n102 = event-data() -> ()  [unwired: 1 in, 3 out]
      }
      event "K", "B", "蠕动泵最小频率(Hz)", "蠕动泵最大频率(Hz)", "加标体积(mL)", "注射泵注出量", "注射泵注入量": Mouse Down {
        n103 = event-data() -> ("CtlRef"=w189:refnum<vi>)  [unwired: 1 in, 2 out]
        n104 = property class="DigNum (严格)"(reference=w189) -> (reference out=w188:refnum<vi>, "Value"=w186:sgl)  [unwired: 1 in, 1 out]
        n105 = call "数字键盘.vi"("OldNumber"=w186) -> ("NewNumber"=w187:sgl)
        n106 = property class="DigNum (严格)"(reference=w188, "Val(Sgnl)"=w187) -> ()  [unwired: 1 in, 2 out]
      }
      event "注射泵注出量", "注射泵注入量": Value Change {
        w191 = sgl 1000.0 ("y")
        n107 = event-data() -> ("CtlRef"=w192:refnum<vi>, "NewVal"=w193:sgl)  [unwired: 1 in, 4 out]
        n108 = Greater Or Equal?(x=w193, y=w191) -> (x >= y?=w190:bool)
        n109 = case shown="真" w190 {
          tunnel: w192 -> [_ w195]
          tunnel: w191 -> [_ w194]
          frame False {
          }
          frame True {
            n110 = property class="DigNum (严格)"(reference=w195, "Value"=w194) -> ()  [unwired: 1 in, 2 out]
          }
        }
      }
      event "注射泵系数读取": Value Change {
        n111 = event-data() -> ()  [unwired: 1 in, 4 out]
        n112 = call "ZK注射泵系数读取.vi"("是否启用通讯通知"=TRUE, "Slave ID"=w196) -> ("error out"=w198:errorcluster, "B"=w199:sgl, "K"=w200:sgl)  [unwired: 7 in]
        n113 = local write "K"(w200) -> ()
        n114 = local write "B"(w199) -> ()
      }
      event "注射泵系数写入": Value Change {
        n115 = event-data() -> ()  [unwired: 1 in, 4 out]
        n116 = call "ZK注射泵系数写入.vi"("是否启用通讯通知"=TRUE, "B"="B", "K"="K", "Slave ID"=w201) -> ("error out"=w203:errorcluster)  [unwired: 7 in]
      }
      event "蠕动泵参数写入": Value Change {
        n117 = event-data() -> ()  [unwired: 1 in, 5 out]
        n118 = call "ZK蠕动泵频率参数写入.vi"("是否启用通讯通知"=TRUE, "蠕动泵最小频率"="蠕动泵最小频率(Hz)", "蠕动泵最大频率"="蠕动泵最大频率(Hz)", "Slave ID"=w206) -> ("error out"=w210:errorcluster)  [unwired: 7 in]
      }
      event "蠕动泵参数读取": Value Change {
        n119 = event-data() -> ()  [unwired: 1 in, 5 out]
        n120 = call "ZK蠕动泵频率参数读取.vi"("是否启用通讯通知"=TRUE, "Slave ID"=w211) -> ("error out"=w213:errorcluster, "蠕动泵最小频率"=w214:i32, "蠕动泵最大频率"=w215:i32)  [unwired: 7 in]
        n121 = local write "蠕动泵最大频率(Hz)"(w215) -> ()
        n122 = local write "蠕动泵最小频率(Hz)"(w214) -> ()
      }
      event "加标体积写入": Value Change {
        n123 = event-data() -> ()  [unwired: 1 in, 6 out]
        n124 = call "ZK加标体积写入.vi"("是否启用通讯通知"=TRUE, "加标体积"="加标体积(mL)", "Slave ID"=w216) -> ("error out"=w219:errorcluster)  [unwired: 8 in]
      }
      event "加标体积读取": Value Change {
        n125 = event-data() -> ()  [unwired: 1 in, 6 out]
        n126 = call "ZK加标体积读取.vi"("是否启用通讯通知"=TRUE, "Slave ID"=w220) -> ("error out"=w223:errorcluster, "加标体积"=w222:sgl)  [unwired: 8 in]
        n127 = local write "加标体积(mL)"(w222) -> ()
      }
      event "三通阀打开": Value Change {
        n128 = event-data() -> ()  [unwired: 1 in, 6 out]
        n129 = call "ZK注射泵操作.vi"("是否启用通讯通知"=TRUE, "注射泵操作"=质控注射泵操作."打开三通阀", "Slave ID"=w224) -> ("error out"=w226:errorcluster)  [unwired: 8 in]
      }
      event "三通阀关闭": Value Change {
        n130 = event-data() -> ()  [unwired: 1 in, 6 out]
        n131 = call "ZK注射泵操作.vi"("是否启用通讯通知"=TRUE, "注射泵操作"=质控注射泵操作."关闭三通阀", "Slave ID"=w228) -> ("error out"=w231:errorcluster)  [unwired: 8 in]
      }
      event "注射泵注入": Value Change {
        n132 = event-data() -> ()  [unwired: 1 in, 6 out]
        n133 = Multiply(x=sgl 2.0, y="注射泵注入量") -> (x*y=w233:sgl)
        n134 = call "ZK注射泵操作.vi"("是否启用通讯通知"=FALSE, "注射泵操作"=质控注射泵操作."关闭三通阀", "Slave ID"=w234) -> ("error out"=w235:errorcluster)  [unwired: 8 in]
        n135 = call "ZK注射泵操作.vi"("是否启用通讯通知"=TRUE, "error in (no error)"=w235, "注射泵操作步"=w233, "注射泵操作"=质控注射泵操作."注射泵吸入", "Slave ID"=w234) -> ("error out"=w241:errorcluster)  [unwired: 6 in]
      }
      event "注射泵注出": Value Change {
        n136 = event-data() -> ()  [unwired: 1 in, 6 out]
        n137 = Multiply(x="注射泵注出量", y=sgl 2.0) -> (x*y=w243:sgl)
        n138 = call "ZK注射泵操作.vi"("是否启用通讯通知"=FALSE, "注射泵操作"=质控注射泵操作."打开三通阀", "Slave ID"=w245) -> ("error out"=w244:errorcluster)  [unwired: 8 in]
        n139 = call "ZK注射泵操作.vi"("是否启用通讯通知"=TRUE, "error in (no error)"=w244, "注射泵操作步"=w243, "注射泵操作"=质控注射泵操作."注射泵排出", "Slave ID"=w245) -> ("error out"=w251:errorcluster)  [unwired: 6 in]
      }
      event "注射泵暂停": Value Change {
        n140 = event-data() -> ()  [unwired: 1 in, 6 out]
        n141 = call "ZK注射泵操作.vi"("是否启用通讯通知"=TRUE, "注射泵操作"=质控注射泵操作."注射泵暂停", "Slave ID"=w252) -> ("error out"=w255:errorcluster)  [unwired: 8 in]
      }
      event "注射泵复位": Value Change {
        n142 = event-data() -> ()  [unwired: 1 in, 6 out]
        n143 = call "ZK注射泵操作.vi"("是否启用通讯通知"=TRUE, "注射泵操作"=质控注射泵操作."注射泵复位", "Slave ID"=w256) -> ("error out"=w259:errorcluster)  [unwired: 8 in]
      }
      event "三通阀1关闭": Value Change {
        w263 = u16 1 items=["打开三通阀", "关闭三通阀"] ("三通阀1操作")
        n144 = event-data() -> ()  [unwired: 1 in, 6 out]
        n145 = call "ZK三通阀1操作.vi"("是否启用通讯通知"=TRUE, "三通阀1操作"=w263, "Slave ID"=w260) -> ("error out"=w262:errorcluster)  [unwired: 8 in]
      }
      event "三通阀1打开": Value Change {
        w267 = u16 0 items=["打开三通阀", "关闭三通阀"] ("三通阀1操作")
        n146 = event-data() -> ()  [unwired: 1 in, 6 out]
        n147 = call "ZK三通阀1操作.vi"("是否启用通讯通知"=TRUE, "三通阀1操作"=w267, "Slave ID"=w264) -> ("error out"=w266:errorcluster)  [unwired: 8 in]
      }
      event "三通阀2打开": Value Change {
        w271 = u16 0 items=["打开三通阀", "关闭三通阀"] ("三通阀2操作")
        n148 = event-data() -> ()  [unwired: 1 in, 6 out]
        n149 = call "ZK三通阀2操作.vi"("是否启用通讯通知"=TRUE, "三通阀2操作"=w271, "Slave ID"=w268) -> ("error out"=w270:errorcluster)  [unwired: 8 in]
      }
      event "三通阀2关闭": Value Change {
        w275 = u16 1 items=["打开三通阀", "关闭三通阀"] ("三通阀2操作")
        n150 = event-data() -> ()  [unwired: 1 in, 6 out]
        n151 = call "ZK三通阀2操作.vi"("是否启用通讯通知"=TRUE, "三通阀2操作"=w275, "Slave ID"=w272) -> ("error out"=w274:errorcluster)  [unwired: 8 in]
      }
      event "蠕动泵1反转": Value Change {
        w278 = T13 3 items=["蠕动泵正转"=2, "蠕动泵反转"=3, "蠕动泵停止"=4] ("蠕动泵1操作")
        n152 = event-data() -> ()  [unwired: 1 in, 6 out]
        n153 = call "ZK蠕动泵1操作.vi"("是否启用通讯通知"=TRUE, "蠕动泵1操作"=w278, "Slave ID"=w276) -> ("error out"=w279:errorcluster)  [unwired: 8 in]
      }
      event "蠕动泵1正转": Value Change {
        w282 = T13 2 items=["蠕动泵正转"=2, "蠕动泵反转"=3, "蠕动泵停止"=4] ("蠕动泵1操作")
        n154 = event-data() -> ()  [unwired: 1 in, 6 out]
        n155 = call "ZK蠕动泵1操作.vi"("是否启用通讯通知"=TRUE, "蠕动泵1操作"=w282, "Slave ID"=w280) -> ("error out"=w283:errorcluster)  [unwired: 8 in]
      }
      event "蠕动泵1停止": Value Change {
        w286 = T13 4 items=["蠕动泵正转"=2, "蠕动泵反转"=3, "蠕动泵停止"=4] ("蠕动泵1操作")
        n156 = event-data() -> ()  [unwired: 1 in, 6 out]
        n157 = call "ZK蠕动泵1操作.vi"("是否启用通讯通知"=TRUE, "蠕动泵1操作"=w286, "Slave ID"=w284) -> ("error out"=w287:errorcluster)  [unwired: 8 in]
      }
      event "蠕动泵2反转": Value Change {
        w290 = T13 3 items=["蠕动泵正转"=2, "蠕动泵反转"=3, "蠕动泵停止"=4] ("蠕动泵2操作")
        n158 = event-data() -> ()  [unwired: 1 in, 6 out]
        n159 = call "ZK蠕动泵2操作.vi"("是否启用通讯通知"=TRUE, "蠕动泵2操作"=w290, "Slave ID"=w288) -> ("error out"=w291:errorcluster)  [unwired: 8 in]
      }
      event "蠕动泵2正转": Value Change {
        w294 = T13 2 items=["蠕动泵正转"=2, "蠕动泵反转"=3, "蠕动泵停止"=4] ("蠕动泵2操作")
        n160 = event-data() -> ()  [unwired: 1 in, 6 out]
        n161 = call "ZK蠕动泵2操作.vi"("是否启用通讯通知"=TRUE, "蠕动泵2操作"=w294, "Slave ID"=w292) -> ("error out"=w295:errorcluster)  [unwired: 8 in]
      }
      event "蠕动泵2停止": Value Change {
        w298 = T13 4 items=["蠕动泵正转"=2, "蠕动泵反转"=3, "蠕动泵停止"=4] ("蠕动泵2操作")
        n162 = event-data() -> ()  [unwired: 1 in, 6 out]
        n163 = call "ZK蠕动泵2操作.vi"("是否启用通讯通知"=TRUE, "蠕动泵2操作"=w298, "Slave ID"=w296) -> ("error out"=w299:errorcluster)  [unwired: 8 in]
      }
      event "组合操作进水样": Value Change {
        n164 = event-data() -> ()  [unwired: 1 in, 6 out]
        n165 = call "ZK组合命令区.vi"("是否启用通讯通知"=TRUE, "组合命令区"=质控组合命令区."进水样", "Slave ID"=w300) -> ("error out"=w303:errorcluster)  [unwired: 8 in]
      }
      event "组合操作排废液": Value Change {
        n166 = event-data() -> ()  [unwired: 1 in, 6 out]
        n167 = call "ZK组合命令区.vi"("是否启用通讯通知"=TRUE, "组合命令区"=质控组合命令区."排废液", "Slave ID"=w304) -> ("error out"=w307:errorcluster)  [unwired: 8 in]
      }
      event "组合操作进空气": Value Change {
        n168 = event-data() -> ()  [unwired: 1 in, 6 out]
        n169 = call "ZK组合命令区.vi"("是否启用通讯通知"=TRUE, "组合命令区"=质控组合命令区."进空气（搅拌）", "Slave ID"=w308) -> ("error out"=w311:errorcluster)  [unwired: 8 in]
      }
      event "组合操作定量": Value Change {
        n170 = event-data() -> ()  [unwired: 1 in, 6 out]
        n171 = call "ZK组合命令区.vi"("是否启用通讯通知"=TRUE, "组合命令区"=质控组合命令区."定量（反转定量）", "Slave ID"=w312) -> ("error out"=w315:errorcluster)  [unwired: 8 in]
      }
      event "组合操作停止": Value Change {
        n172 = event-data() -> ()  [unwired: 1 in, 6 out]
        n173 = call "ZK组合命令区.vi"("是否启用通讯通知"=TRUE, "组合命令区"=质控组合命令区."停止", "Slave ID"=w316) -> ("error out"=w319:errorcluster)  [unwired: 8 in]
      }
      event "启动进样流程": Value Change {
        n174 = event-data() -> ()  [unwired: 1 in, 6 out]
        n175 = call "ZK流程控制.vi"("是否启用通讯通知"=TRUE, "流程控制"=质控流程控制."启动进样流程", "Slave ID"=w320) -> ("error out"=w323:errorcluster)  [unwired: 8 in]
      }
      event "启动加标流程": Value Change {
        n176 = event-data() -> ()  [unwired: 1 in, 6 out]
        n177 = call "ZK流程控制.vi"("是否启用通讯通知"=TRUE, "流程控制"=质控流程控制."启动加标流程", "Slave ID"=w324) -> ("error out"=w327:errorcluster)  [unwired: 8 in]
      }
      event "启动排液流程": Value Change {
        n178 = event-data() -> ()  [unwired: 1 in, 6 out]
        n179 = call "ZK流程控制.vi"("是否启用通讯通知"=TRUE, "流程控制"=质控流程控制."启动排液流程", "Slave ID"=w328) -> ("error out"=w331:errorcluster)  [unwired: 8 in]
      }
      event "停止所有流程": Value Change {
        n180 = event-data() -> ()  [unwired: 1 in, 6 out]
        n181 = call "ZK流程控制.vi"("是否启用通讯通知"=TRUE, "流程控制"=质控流程控制."停止流程", "Slave ID"=w332) -> ("error out"=w335:errorcluster)  [unwired: 8 in]
      }
      event "启动水样润洗流程": Value Change {
        n182 = event-data() -> ()  [unwired: 1 in, 6 out]
        n183 = call "ZK流程控制.vi"("是否启用通讯通知"=TRUE, "流程控制"=质控流程控制."启动水样润洗流程", "Slave ID"=w336) -> ("error out"=w339:errorcluster)  [unwired: 8 in]
      }
      event "启动加标润洗流程": Value Change {
        n184 = event-data() -> ()  [unwired: 1 in, 6 out]
        n185 = call "ZK流程控制.vi"("是否启用通讯通知"=TRUE, "流程控制"=质控流程控制."启动加标润洗流程", "Slave ID"=w340) -> ("error out"=w343:errorcluster)  [unwired: 8 in]
      }
    }
  }
  n186 = property on="Tab Control 3" class="TabCtl (严格)"("Visible"=w1) -> ("Visible"=w8:bool)  [unwired: 2 in, 2 out]
  n187 = property class="App"() -> ("Disp.WkSpace"=w6:T14)  [unwired: 2 in, 2 out]
  n188 = Select(t=T5 {"Left"=744, "Top"=804} ("位置"), s=w8, f=T5 {"Left"=744, "Top"=432} ("位置")) -> (s? t:f=w10:T5)
  n189 = Select(t=T5 {"Left"=900, "Top"=880} ("位置"), s=w8, f=T5 {"Left"=900, "Top"=500} ("位置")) -> (s? t:f=w5:T5)
  n190 = property on="关闭" class="Bool"("Position"=w10) -> ()  [unwired: 2 in, 2 out]
  n191 = call "取中心点.vi"("前面板窗口:最小尺寸"=w5, "显示:主工作区"=w6) -> ("前面板窗口:窗口边界"=w4:T14)  [unwired: 9 in]
  n192 = control-ref of="本VI"() -> (w3:refnum<vi>)
  n193 = property class="VI"(reference=w3, "Front Panel.PanelBounds"=w4) -> ()  [unwired: 1 in, 2 out]
